vi "Unflatten LIBN.vi"(8 "error in (no error)":errorcluster, 11 "Data in":string) -> (0 "error out":errorcluster, 2 "Libraries (MD5 Salt)":string, 3 "Owning Libraries (*.lvlib, *.lvclass)":string[](array[string]))   [LabVIEW 2018, in "VI-Hacker.lvlib"]
uses:
  VI-Hacker.lvlib
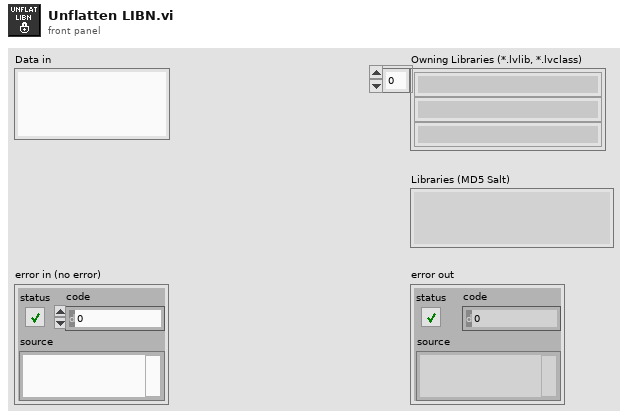
[diagram p1: front panel]
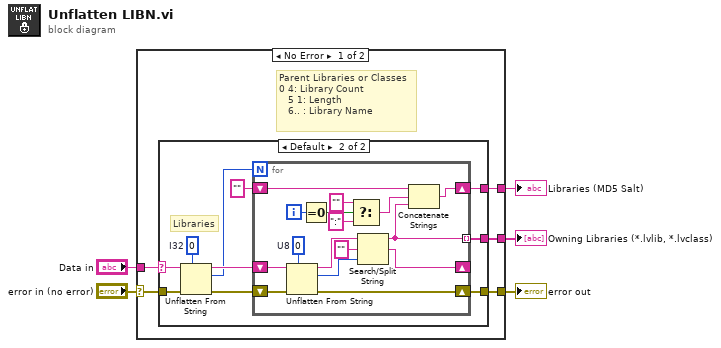
[diagram p0: block diagram]
diagram:
  n1 = case shown="No Error" "error in (no error)" {
    selector: "error in (no error)" -> [w9 w38]
    tunnel: "Data in" -> [w6 _]
    tunnel: [w10 _] -> w4
    tunnel: [w8 w38] -> w2
    tunnel: [w7 _] -> w1
    frame No Error {
      # "Parent Libraries or Classes\n0 4: Library Count\n   5 1: Length\n   6.. : Library Name"
      n2 = case shown="Default" w6 {
        selector: w6 -> [_ w12]
        tunnel: [_ w21] -> w10
        tunnel: w9 -> [w11 w16]
        tunnel: [w11 w15] -> w8
        tunnel: [_ w13] -> w7
        frame "" {
          # "Not part of a library"
        }
        frame Default {
          w20 = 0  # I32
          # "Libraries"
          n3 = Unflatten From String(type=w20, binary string=w12, error in (no error)=w16) -> (rest of the binary string=w18:string, value=w17:i32, error out=w19:errorcluster)  [unwired: 2 in]
          n4 = for {
            N: w17 -> [_]
            shift-right: [w30] -> _
            shift-left: w18 -> [w35]
            shift-right: [w31] -> w15
            shift-left: w19 -> [w36]
            tunnel: [w22] -> w21 mode=indexing
            shift-right: [w24] -> w13
            shift-left: "" -> [w25]
            i -> [w29]
            w37 = u8 0  # U8
            n5 = Unflatten From String(type=w37, binary string=w35, error in (no error)=w36) -> (rest of the binary string=w34:string, value=w33:u8, error out=w31:errorcluster)  [unwired: 2 in]
            n6 = Equal To 0?(x=w29) -> (x = 0?=w28:bool)
            n7 = Select(t="", s=w28, f=":") -> (s? t:f=w23:string)
            n8 = Search/Split String(string=w34, search string/char (-)="", offset (0)=w33) -> (substring before match=w22:string, match + rest of string=w30:string)  [unwired: 1 out]
            n9 = Concatenate Strings(w25, w23, w22) -> (w24:string)
          }
        }
      }
    }
    frame Error {
    }
  }
  "error out" <- w2
  "Owning Libraries (*.lvlib, *.lvclass)" <- w4
  "Libraries (MD5 Salt)" <- w1
